vi "Create Components DVR.vi"(8 "error in (no error)":errorcluster, 11 "Item Ref in":T1 format="%.0x") -> (0 "error out":errorcluster, 3 "Item Ref out":T1 format="%.0x")   [LabVIEW 2017, in "DSF System Explorer.lvlib"]
uses:
  DSF System Explorer.lvlib
  <vilib>/NI Veristand/Custom Device API/Custom Device Item Ref.ctl
  Components.ctl
  DSF Core.lvlibp/Classes/Component/Component.lvclass
  <vilib>/NI Veristand/Custom Device API/Set Item Property (U32).vi
  <vilib>/NI Veristand/Custom Device API/Custom Device API.lvlib
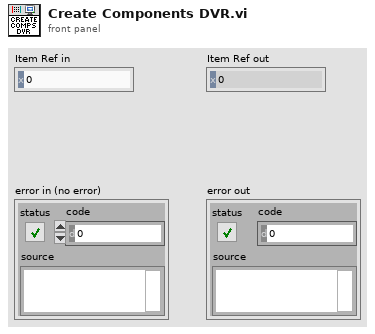
[diagram p1: front panel]
types:
  T1 = typedef "Custom Device API.lvlib/Custom Device Item Ref.ctl" = u64
  T2 = typedef "DSF System Explorer.lvlib/Components.ctl" = cluster{"Components":refnum<class "Component.lvclass">[]}
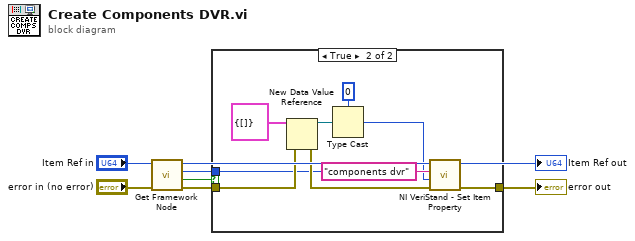
[diagram p0: block diagram]
diagram:
  n1 = call "Get Framework Node.vi"("error in (no error)"="error in (no error)", "Item Ref in"="Item Ref in") -> ("error out"=w5:errorcluster, "found?"=w2:bool, "Framework Ref"=w4:T1, "Item Ref out"=→"Item Ref out":T1)  [unwired: 6 in]
  n2 = case shown="True" w2 {
    tunnel: w5 -> [w8 w12]
    tunnel: w4 -> [_ w9]
    tunnel: [w8 w16] -> w3
    frame False {
    }
    frame True {
      n3 = New Data Value Reference(data value=T2 {"Components"=[]}, error in=w12) -> (data value reference=w10:refnum<data-value>, error out=w11:errorcluster)
      n4 = Type Cast(type=u32 0, x=w10) -> (*(type *) &x=w14:u32)
      n5 = call-poly <vilib>:"NI VeriStand - Set Item Property.vi"("error in (no error)"=w11, "Value"=w14, "Property Name"="components dvr", "Item Ref in"=w9) -> ("error out"=w16:errorcluster)  [unwired: 5 in, 2 out]
    }
  }
  "error out" <- w3
